vi "InitProperties.vi"(0 "reference":refnum<k24>) -> ()   [LabVIEW 2019, in "XTextCode.xctl"]
uses:
  XTextCode.xctl
  System.Windows.Forms
  System.Drawing
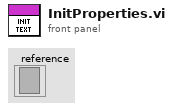
[diagram p1: front panel]
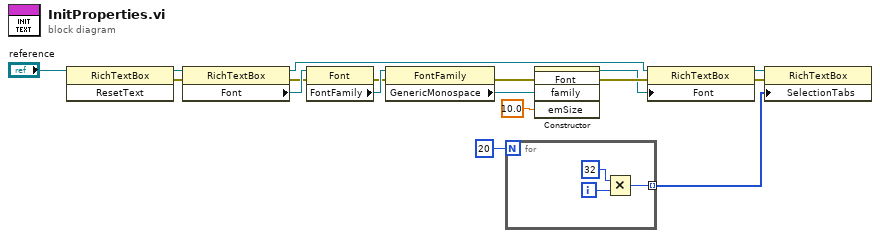
[diagram p0: block diagram]
diagram:
  n1 = invoke class="RichTextBox" method="ResetText"(reference="reference") -> (reference out=w17:refnum<k24>, error out=w10:errorcluster)  [unwired: 2 in, 1 out]
  n2 = property class="RichTextBox"(reference=w17, error in=w10) -> (reference out=w1:refnum<k24>, error out=w9:errorcluster, "Font"=w16:refnum<k24>)
  n3 = property class="Font"(reference=w16, error in=w9) -> (error out=w8:errorcluster, "FontFamily"=w15:refnum<k24>)  [unwired: 1 out]
  n4 = property class="FontFamily"(reference=w15, error in=w8) -> (error out=w7:errorcluster, "GenericMonospace"=w14:refnum<k24>)  [unwired: 1 out]
  n5 = for {
    N: 20 -> [_]
    tunnel: [w18] -> w4 mode=indexing
    i -> [w20]
    n6 = Multiply(x=32, y=w20) -> (x*y=w18:i32)
  }
  n7 = constructor class="Font"(error in=w7, "family"=w14, "emSize"=sgl 10.0) -> (reference out=w2:refnum<k24>, error out=w6:errorcluster)  [unwired: 2 in, 3 out]
  n8 = property class="RichTextBox"(reference=w1, error in=w6, "Font"=w2) -> (reference out=w11:refnum<k24>, error out=w12:errorcluster)
  n9 = property class="RichTextBox"(reference=w11, error in=w12, "SelectionTabs"=w4) -> ()  [unwired: 2 out]
